vi "ClearEventsTDC.vi"(8 "error in (no error)":errorcluster, 10 "handle":i32, 11 "VME module Base Address":u32) -> (0 "error out":errorcluster, 2 "VME module Base Address out":u32, 3 "handle out":i32)   [LabVIEW 2014]
uses:
  Program Files (x86)/CAEN/Comm/labview/CAENComm.lvlib
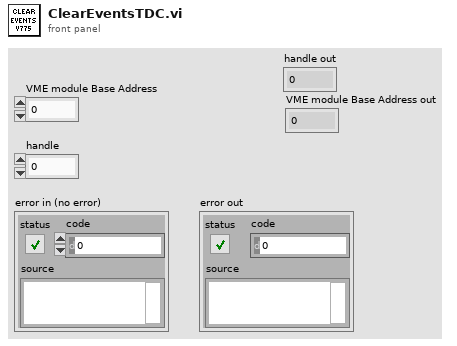
[diagram p1: front panel]
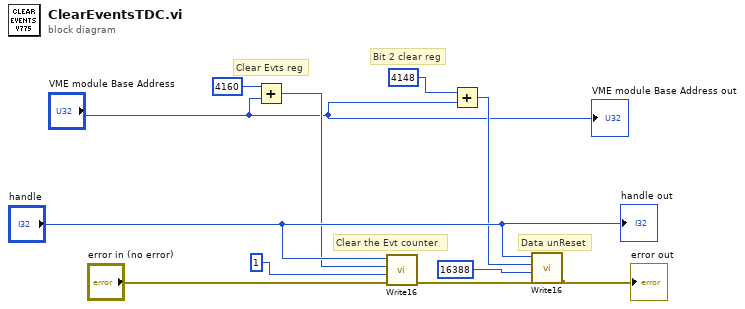
[diagram p0: block diagram]
diagram:
  # "Bit 2 clear reg"
  # "Data unReset"
  # "Clear Evts reg"
  # "Clear the Evt counter"
  n1 = Add(x=u32 4160, y="VME module Base Address") -> (x+y=w3:u32)
  n2 = call "Write16.vi"("error in (no error)"="error in (no error)", "Data"=u16 1, "Address"=w3, "handle"="handle") -> ("error out"=w6:errorcluster)  [unwired: 7 in]
  n3 = Add(x=u32 4148, y="VME module Base Address") -> (x+y=w10:u32)
  n4 = call "Write16.vi"("error in (no error)"=w6, "Data"=u16 16388, "Address"=w10, "handle"="handle") -> ("error out"=→"error out":errorcluster)  [unwired: 7 in]
  "handle out" <- "handle"
  "VME module Base Address out" <- "VME module Base Address"
